vi "弹窗-提示选择Com口-30.vi"(7 "存储间隔（小时）":dbl=1.0 min=0.5, 8 "VI引用句柄":refnum<vi>, 9 "实时数据列表":refnum<vi>, 10 "测量值":cluster{"X":timestamp, "Y":dbl}[](array[cluster]), 11 "暂停发送-引用":refnum<vi>) -> (3 "存储间隔（h）":dbl=1.0 min=1.0)   [LabVIEW 2017]
uses:
  <vilib>/Utility/xml.llb/Write to XML File(string).vi
panel:
  in  "联系人数组":cluster{"姓名":string, "手机号":string}[](array[cluster])
  in  "通讯录菜单":enum16{"添加", "删除"}(ring)
  in  "确定":bool
  in  "取消":bool
  in  "选项卡控件":enum32{"通信设置", "短信通知", "调试选项"}(tab)
  in  "静音与恢复延迟（秒）":u16=1 min=1
  in  "VISA资源名称":refnum<visa-resource-name> caption="通信串口"
  in  "最大探头数":u8=1 min=1 max=32
  in  "波特率":enum16{"9600", "19200"}(ring)
  in  "检查并重置33号":bool caption="btn_微调"
  out "重置33号结果":string
  in  "密码":string
  in  "短信通道":string
  in  "员工编号":string
  in  "企业编号":string
  in  "通讯录":i32(listbox)
  in  "添加联系人":bool
  in  "探头地址":u8=1 min=1 max=1 step=1
  in  "N2":u16
  in  "N1":u16
  in  "btn_修改系数":bool
  in  "btn_微调":bool
  in  "微调大小":dbl caption="μSv/h"
  in  "微调模式":enum16{"减小", "增加"}(ring) caption="模式"
  in  "btn_改波特率":bool
  in  "修改波特率":enum16{"9600", "19200"}(ring)=enum."19200"
  # "通信信息"
  # "累积剂量"
  # "通信端口"
  # "波特率"
  # "报警静音"
  # "扫描探头数"
  # "检查隐藏探头"
  # "33号探头作为修改地址所用的临时交接地址 , 修改地址过程异常可能导致探头落入此地址 , \n1. 使用的当前通讯波特率\n2. 实时通信稳定后可设置"
  # "登录信息"
  # "通讯录"
  # "* 短信通知功能需用户自行开通，详询对接平台 http://www.c123.com/"
  # "* 通讯录表格中右键菜单添加或删除联系人"
  # "广播修改波特率"
  # "针对性修改"
  # "测量值微调（μSv/h）"
  # "计算系数"
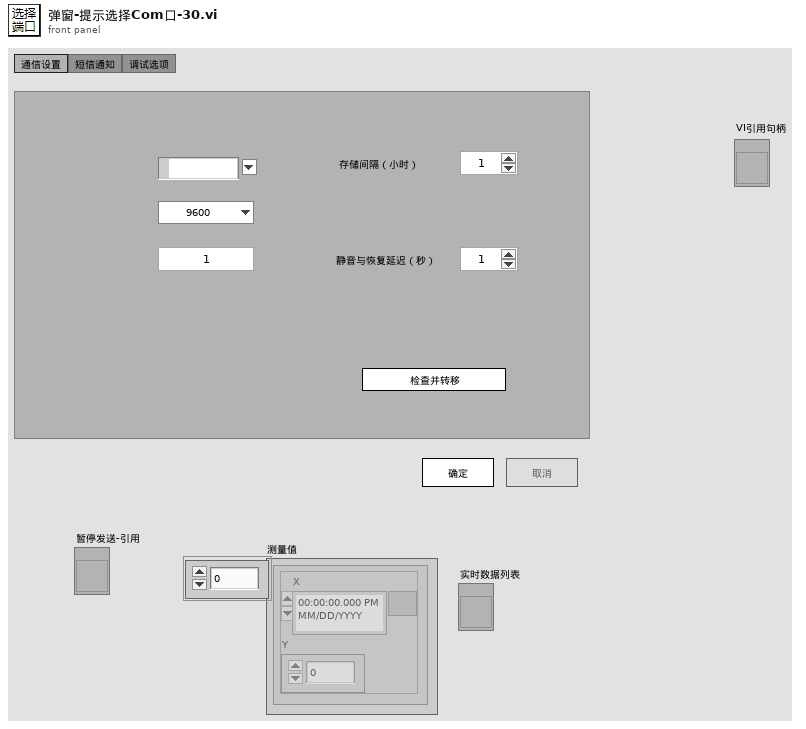
[diagram p1: front panel]
types:
  T1 = enum8{"Enabled", "Disabled", "Disabled and Grayed Out"}
  T2 = enum32{"Invalid", "Standard", "Closed", "Hidden", "Minimized", "Maximized"}
  T3 = enum32{"Page Enabled", "Page Disabled", "Page Disabled & Grayed"}
  T4 = cluster{"企业编号":string, "员工编号":string, "通道号":string, "密码":string, "联系人数组":cluster{"姓名":string, "手机号":string}[]}
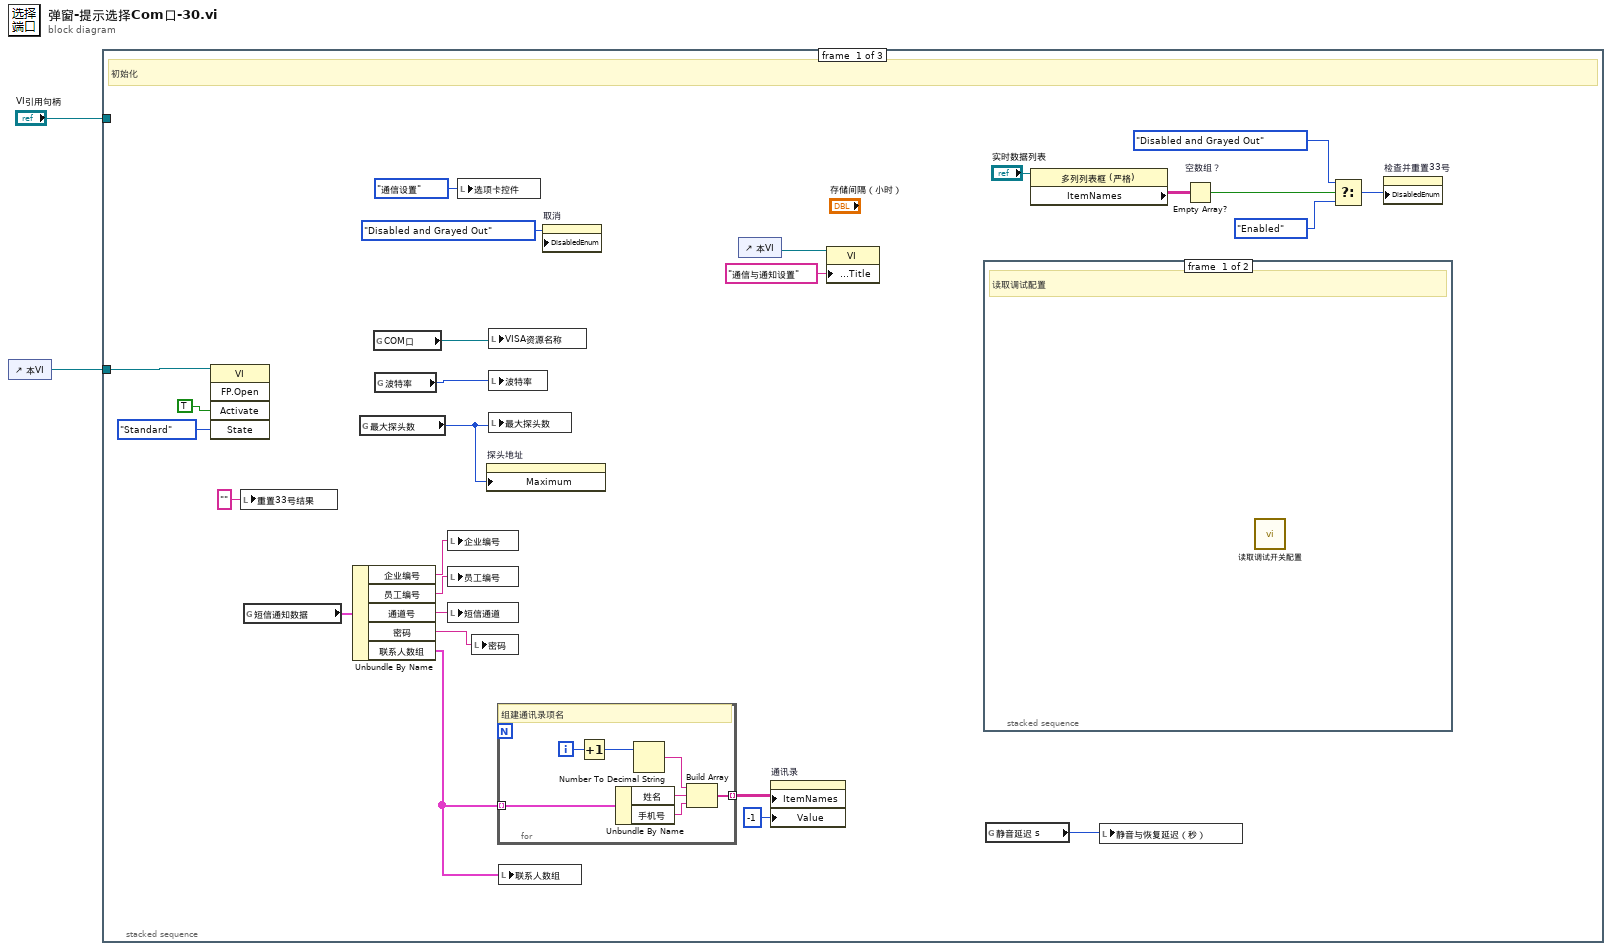
[diagram p0: block diagram]
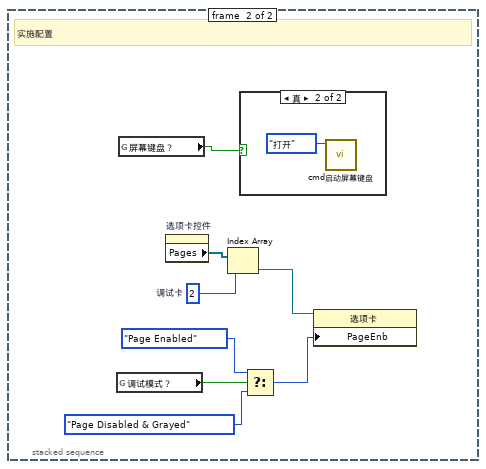
[diagram p2: hidden frame]
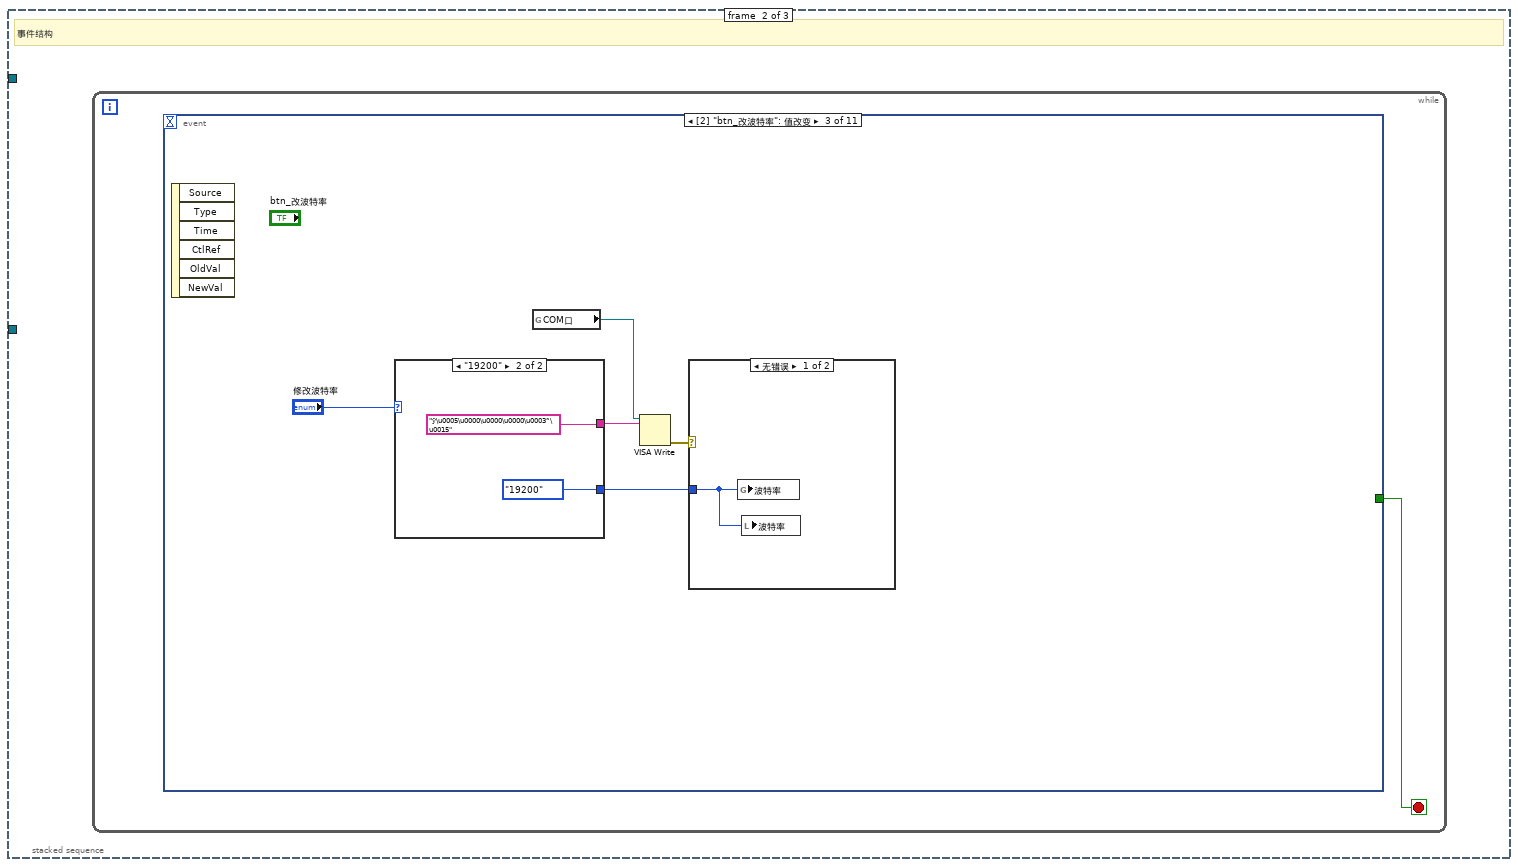
[diagram p4: hidden frame]
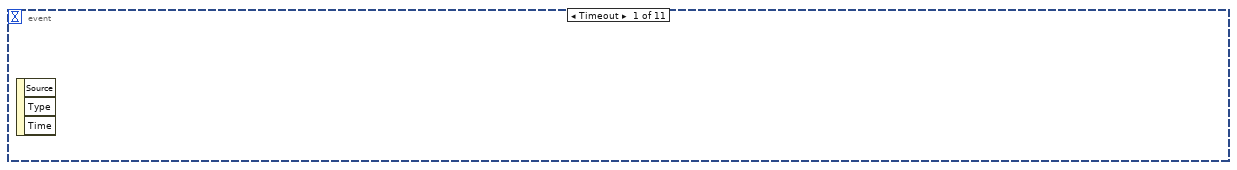
[diagram p5: hidden frame]
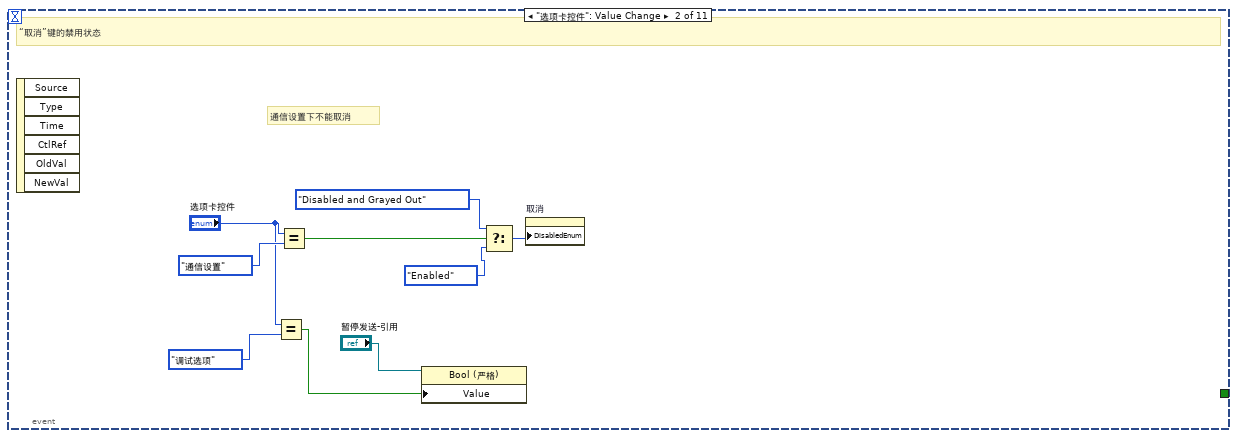
[diagram p6: hidden frame]
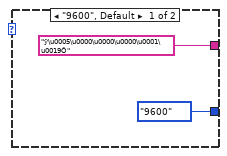
[diagram p8: hidden frame]
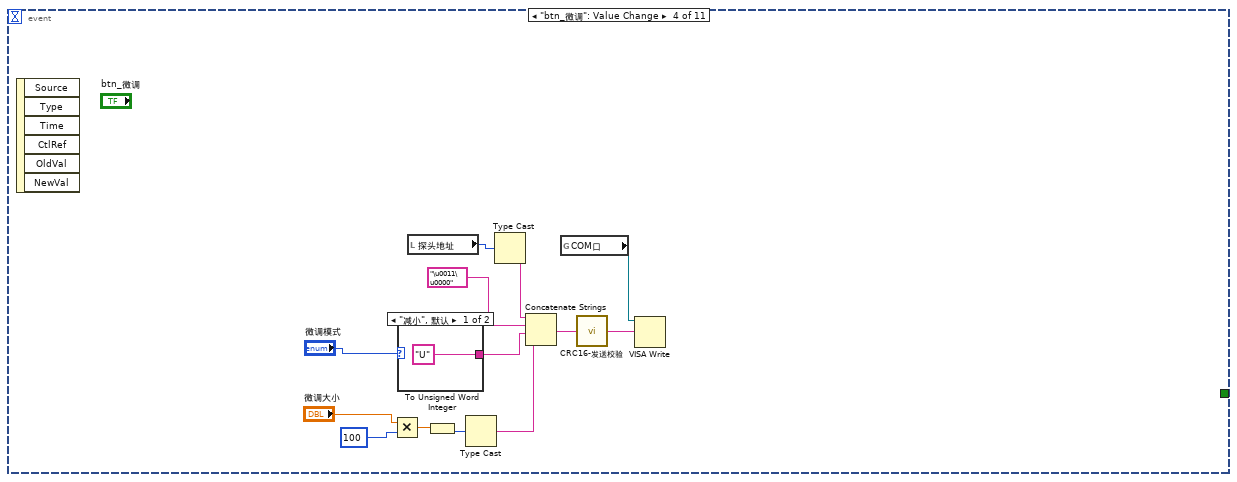
[diagram p9: hidden frame]
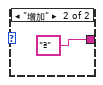
[diagram p10: hidden frame]
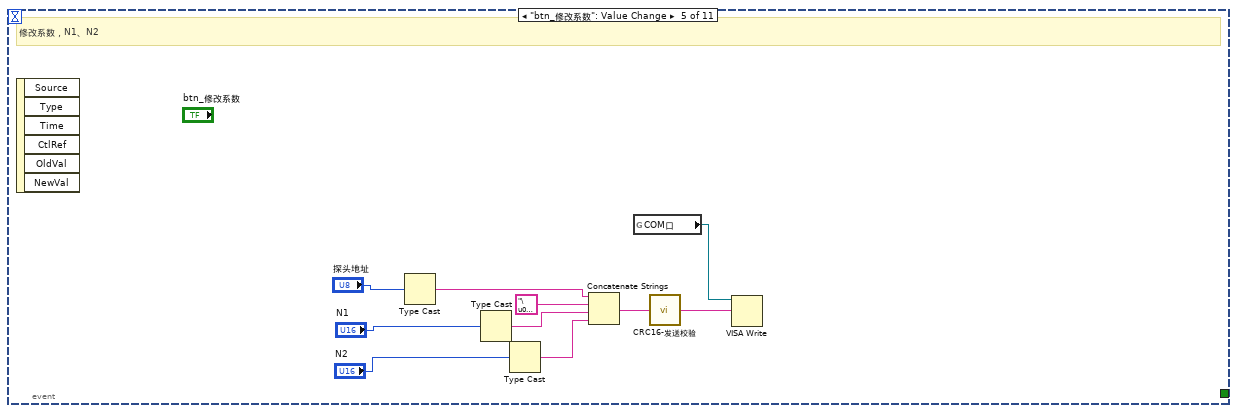
[diagram p11: hidden frame]
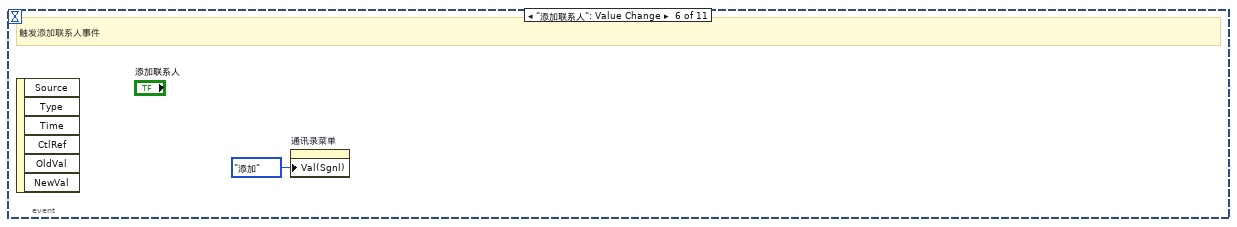
[diagram p12: hidden frame]
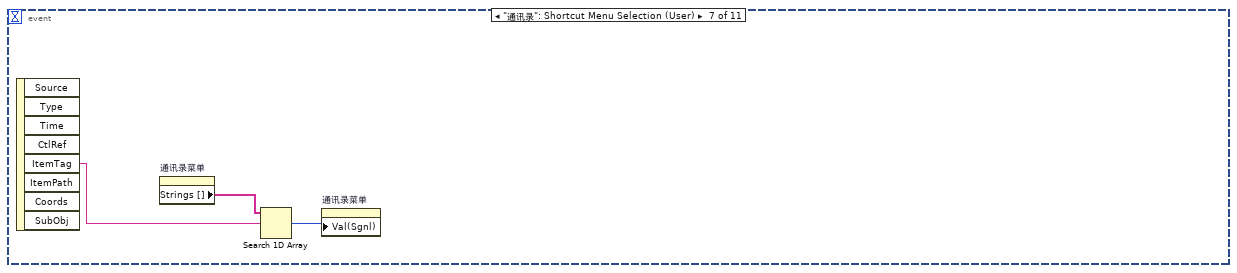
[diagram p13: hidden frame]
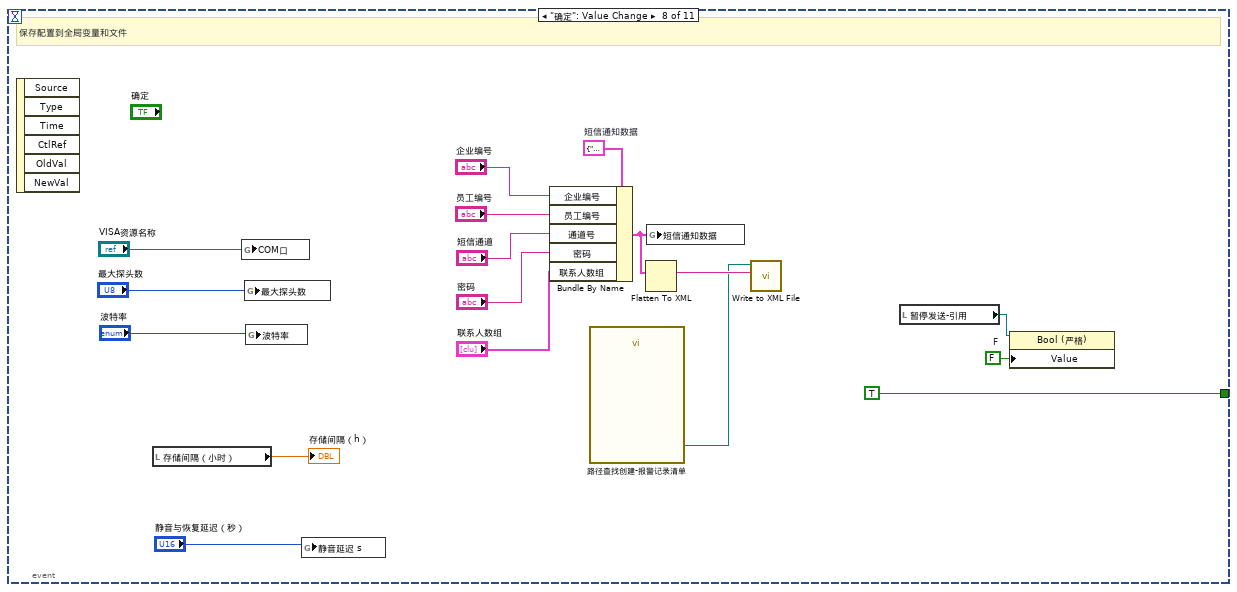
[diagram p14: hidden frame]
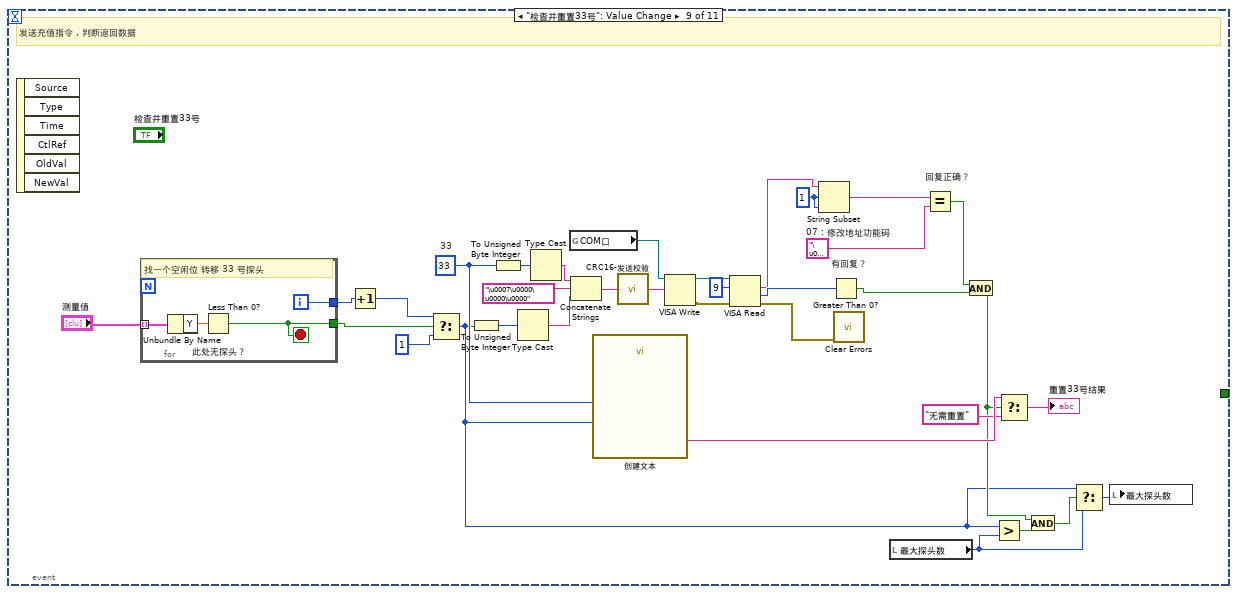
[diagram p15: hidden frame]
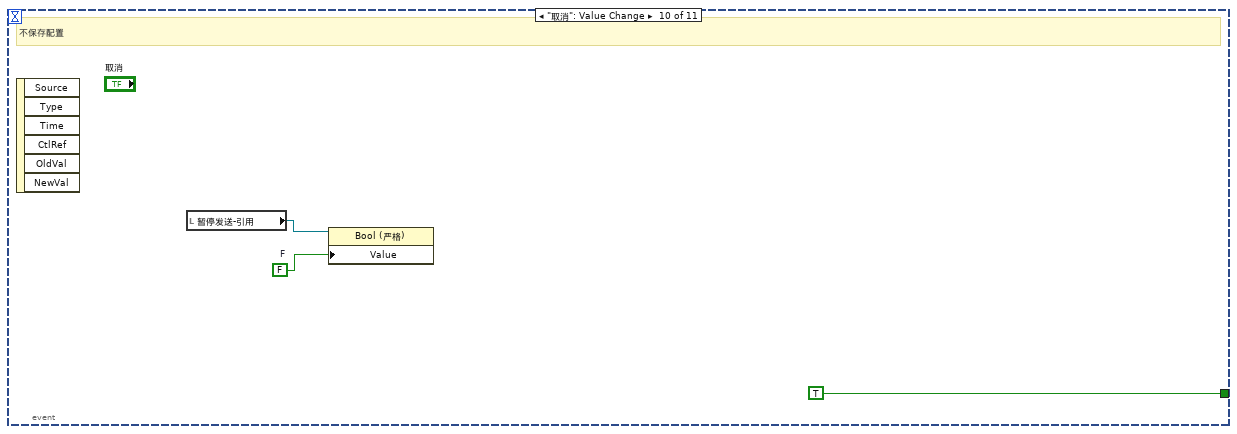
[diagram p16: hidden frame]
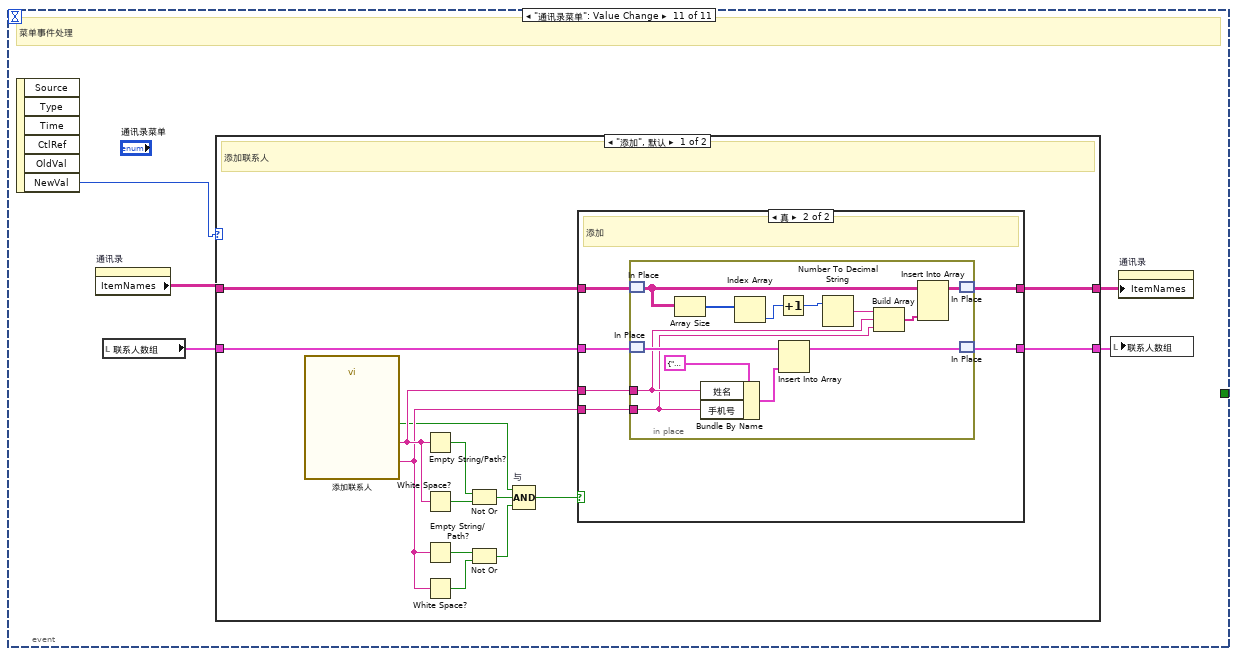
[diagram p17: hidden frame]
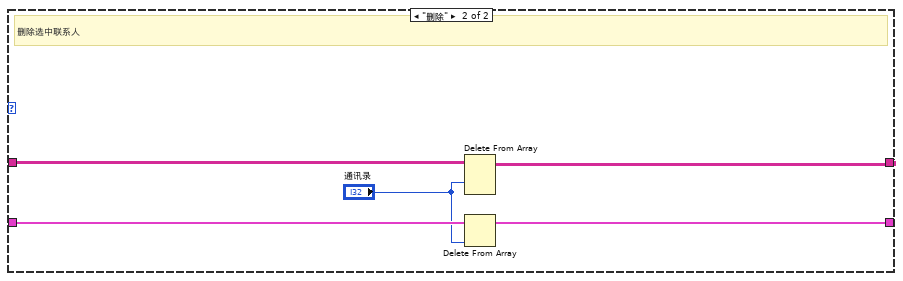
[diagram p19: hidden frame]
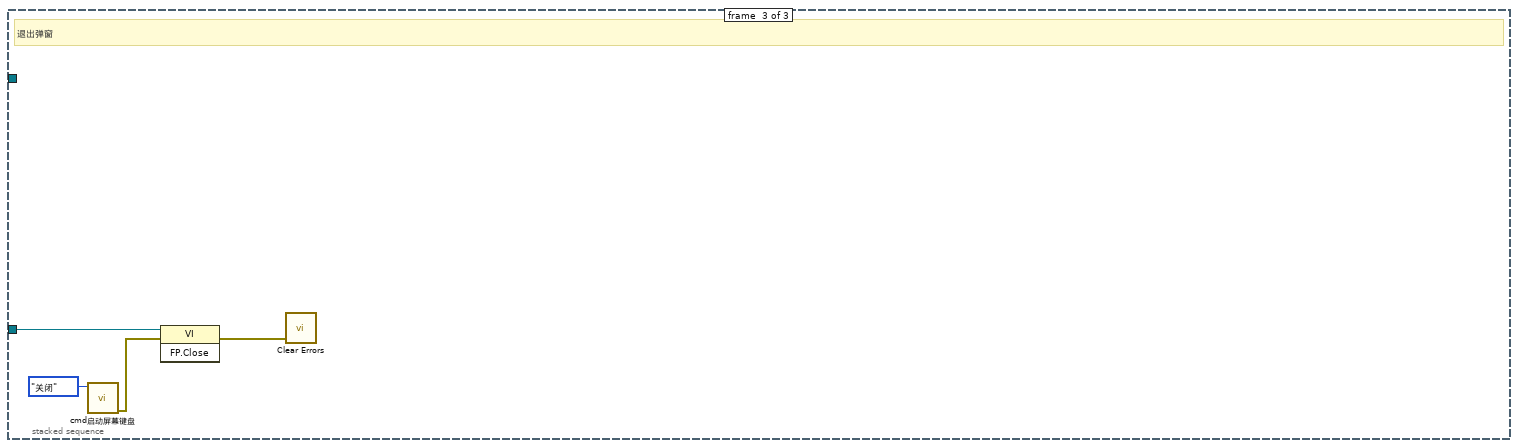
[diagram p20: hidden frame]
diagram:
  n1 = control-ref of="本VI"() -> (w1:refnum<vi>)
  n2 = stacked-sequence {
    tunnel: "VI引用句柄" -> [_ _ _]
    tunnel: w1 -> [w28 _ w200]
    frame #0 {
      # "初始化"
      n3 = invoke class="VI" method="FP.Open"(reference=w28, "Activate"=TRUE ("激活？"), "State"=T2."Standard" ("状态")) -> ()  [unwired: 2 in, 5 out]
      n4 = local write "重置33号结果"("" ("重置33号结果")) -> ()
      n5 = global read "全局变量-35点监测.vi" "短信通知数据"() -> (w19:T4)
      n6 = Unbundle By Name(w19) -> ("企业编号"=w18:string, "员工编号"=w17:string, "通道号"=w16:string, "密码"=w15:string, "联系人数组"=w14:cluster{"姓名":string, "手机号":string}[])
      n7 = global read "全局变量-35点监测.vi" "最大探头数"() -> (w11:i32)
      n8 = global read "全局变量-35点监测.vi" "COM口"() -> (w25:refnum<visa-resource-name>)
      n9 = global read "全局变量-35点监测.vi" "波特率"() -> (w24:enum16{"9600", "19200"})
      n10 = local write "企业编号"(w18) -> ()
      n11 = local write "员工编号"(w17) -> ()
      n12 = local write "短信通道"(w16) -> ()
      n13 = local write "选项卡控件"(enum32{"通信设置", "短信通知"}."通信设置" ("选项卡控件")) -> ()
      n14 = local write "密码"(w15) -> ()
      n15 = property on="探头地址" class="数字 (严格)"("Maximum"=w11) -> ()  [unwired: 2 in, 2 out]
      n16 = local write "VISA资源名称"(w25) -> ()
      n17 = local write "波特率"(w24) -> ()
      n18 = local write "最大探头数"(w11) -> ()
      n19 = for {
        tunnel: w14 -> [w44] mode=indexing
        tunnel: [w41] -> w13 mode=indexing
        i -> [w40]
        # "组建通讯录项名"
        n20 = Increment(x=w40) -> (x+1=w38:i32)
        n21 = Unbundle By Name(w44) -> ("姓名"=w43:string, "手机号"=w42:string)
        n22 = Number To Decimal String(number=w38) -> (decimal integer string=w39:string)  [unwired: 1 in]
        n23 = Build Array(w39, w43, w42) -> (w41:string[])
      }
      n24 = local write "联系人数组"(w14) -> ()
      n25 = property on="取消" class="Bool"("DisabledEnum"=T1."Disabled and Grayed Out" ("禁用")) -> ()  [unwired: 2 in, 2 out]
      n26 = control-ref of="本VI"() -> (w23:refnum<vi>)
      n27 = property on="通讯录" class="MCListbox (严格)"("ItemNames"=w13, "Value"=-1 ("通讯录")) -> ()  [unwired: 2 in, 2 out]
      n28 = property class="VI"(reference=w23, "Front Panel.Title"="通信与通知设置" ("前面板窗口:标题")) -> ()  [unwired: 1 in, 2 out]
      n29 = stacked-sequence {
        frame #0 {
          # "读取调试配置"
          n30 = call "读取调试开关配置.vi"() -> ()  [unwired: 9 in, 3 out]
        }
        frame #1 {
          w35 = 2  # 调试卡
          # "实施配置"
          n31 = global read "全局变量-35点监测.vi" "调试模式？"() -> (w33:bool)
          n32 = global read "全局变量-35点监测.vi" "屏幕键盘？"() -> (w29:bool)
          n33 = property on="选项卡控件" class="选项卡控件 (严格)"() -> ("Pages"=w36:refnum<vi>[])  [unwired: 2 in, 2 out]
          n34 = Index Array(array=w36, index=w35) -> (element=w34:refnum<vi>)
          n35 = case shown="真" w29 {
            frame False {
            }
            frame True {
              n36 = call "cmd启动屏幕键盘.vi"("软键盘开关"=enum16{"关闭", "打开"}."打开") -> ()  [unwired: 9 in, 2 out]
            }
          }
          n37 = Select(t=T3."Page Enabled" ("选项卡页启用状态"), s=w33, f=T3."Page Disabled & Grayed" ("选项卡页启用状态")) -> (s? t:f=w30:T3)
          n38 = property class="选项卡"(reference=w34, "PageEnb"=w30) -> ()  [unwired: 1 in, 2 out]
        }
      }
      n39 = global read "全局变量-35点监测.vi" "静音延迟 s"() -> (w10:u16)
      n40 = property class="多列列表框 (严格)"(reference="实时数据列表") -> ("ItemNames"=w7:string[][])  [unwired: 1 in, 2 out]
      n41 = local write "静音与恢复延迟（秒）"(w10) -> ()
      n42 = Empty Array? "空数组？"(array=w7) -> (empty?=w6:bool)
      n43 = Select(t=T1."Disabled and Grayed Out" ("禁用"), s=w6, f=T1."Enabled" ("禁用")) -> (s? t:f=w3:T1)
      n44 = property on="检查并重置33号" class="Bool"("DisabledEnum"=w3) -> ()  [unwired: 2 in, 2 out]
    }
    frame #1 {
      # "事件结构"
      n45 = while {
        stop <- w45 stop-if-true
        n46 = event shown="[2] \"btn_改波特率\": 值改变" {
          selector: _ -> [_ _ _ _ _ _ _ _ _ _ _]
          dyn-events: _ -> [_ _ _ _ _ _ _ _ _ _ _]
          timeout: _ -> [_ _ _ _ _ _ _ _ _ _ _]
          tunnel: [_ _ _ _ _ _ _ TRUE ("T") _ TRUE ("T") _] -> w45
          event Timeout {
            n47 = event-data() -> ()  [unwired: 1 in, 3 out]
          }
          event "选项卡控件": Value Change {
            # "通信设置下不能取消"
            # "“取消”键的禁用状态"
            n48 = event-data() -> ()  [unwired: 1 in, 6 out]
            n49 = Equal?(x="选项卡控件", y=enum32{"通信设置", "短信通知", "调试选项"}."调试选项" ("选项卡控件")) -> (x = y?=w46:bool)
            n50 = Equal?(x="选项卡控件", y=enum32{"通信设置", "短信通知", "调试选项"}."通信设置" ("选项卡控件")) -> (x = y?=w53:bool)
            n51 = property on="属性节点" class="Bool (严格)"(reference="暂停发送-引用", "Value"=w46) -> ()  [unwired: 1 in, 2 out]
            n52 = Select(t=T1."Disabled and Grayed Out" ("禁用"), s=w53, f=T1."Enabled" ("禁用")) -> (s? t:f=w50:T1)
            n53 = property on="取消" class="Bool"("DisabledEnum"=w50) -> ()  [unwired: 2 in, 2 out]
          }
          event "btn_改波特率": Value Change {
            n54 = event-data() -> ()  [unwired: 1 in, 6 out]
            n55 = case shown="\"19200\"" "修改波特率" {
              tunnel: ["ÿ\u0005\u0000\u0000\u0000\u0001\u0019Ô" "ÿ\u0005\u0000\u0000\u0000\u0003˜\u0015"] -> w57
              tunnel: [enum16{"9600", "19200"}."9600" ("波特率") enum16{"9600", "19200"}."19200" ("波特率")] -> w55
              frame "9600", Default {
              }
              frame "19200" {
              }
            }
            n56 = global read "全局变量-35点监测.vi" "COM口"() -> (w58:refnum<visa-resource-name>)
            n57 = VISA Write(VISA resource name=w58, write buffer=w57) -> (error out=w56:errorcluster)  [unwired: 1 in, 2 out]
            n58 = case shown="无错误" w56 {
              tunnel: w55 -> [w60 _]
              frame No Error {
                n59 = global write "全局变量-35点监测.vi" "波特率"(w60) -> ()
                n60 = local write "波特率"(w60) -> ()
              }
              frame Error {
              }
            }
          }
          event "btn_微调": Value Change {
            n61 = event-data() -> ()  [unwired: 1 in, 6 out]
            n62 = Multiply(x="微调大小", y=100) -> (x*y=w76:dbl)
            n63 = case shown="\"减小\", 默认" "微调模式" {
              tunnel: ["U" "ª"] -> w69
              frame "减小", Default {
              }
              frame "增加" {
              }
            }
            n64 = local read "探头地址"() -> (w72:u8)
            n65 = To Unsigned Word Integer(number=w76) -> (unsigned 16bit integer=w77:u16)
            n66 = Type Cast(x=w77) -> (*(type *) &x=w68:string)  [unwired: 1 in]
            n67 = Type Cast(x=w72) -> (*(type *) &x=w71:string)  [unwired: 1 in]
            n68 = Concatenate Strings(w71, "\u0011\u0000", w69, w68) -> (w67:string)
            n69 = global read "全局变量-35点监测.vi" "COM口"() -> (w65:refnum<visa-resource-name>)
            n70 = call "CRC16-发送校验.vi"("净数据"=w67) -> ("完整输出"=w66:string)
            n71 = VISA Write(VISA resource name=w65, write buffer=w66) -> ()  [unwired: 1 in, 3 out]
          }
          event "btn_修改系数": Value Change {
            # "修改系数，N1、N2"
            n72 = event-data() -> ()  [unwired: 1 in, 6 out]
            n73 = Type Cast(x="探头地址") -> (*(type *) &x=w82:string)  [unwired: 1 in]
            n74 = Type Cast(x="N1") -> (*(type *) &x=w87:string)  [unwired: 1 in]
            n75 = Type Cast(x="N2") -> (*(type *) &x=w85:string)  [unwired: 1 in]
            n76 = Concatenate Strings(w82, "\u0012", w87, w85) -> (w84:string)
            n77 = global read "全局变量-35点监测.vi" "COM口"() -> (w88:refnum<visa-resource-name>)
            n78 = call "CRC16-发送校验.vi"("净数据"=w84) -> ("完整输出"=w89:string)
            n79 = VISA Write(VISA resource name=w88, write buffer=w89) -> ()  [unwired: 1 in, 3 out]
          }
          event "添加联系人": Value Change {
            # "触发添加联系人事件"
            n80 = event-data() -> ()  [unwired: 1 in, 6 out]
            n81 = property on="通讯录菜单" class="Enum (严格)"("Val(Sgnl)"=enum16{"添加", "删除"}."添加" ("值(信号)")) -> ()  [unwired: 2 in, 2 out]
          }
          event "通讯录": Shortcut Menu Selection (User) {
            n82 = event-data() -> ("ItemTag"=w92:string)  [unwired: 1 in, 7 out]
            n83 = property on="通讯录菜单" class="Enum (严格)"() -> ("Strings []"=w93:string[])  [unwired: 2 in, 2 out]
            n84 = Search 1D Array(1D array=w93, element=w92) -> (index of element=w91:i32)  [unwired: 1 in]
            n85 = property on="通讯录菜单" class="Enum (严格)"("Val(Sgnl)"=w91) -> ()  [unwired: 2 in, 2 out]
          }
          event "确定": Value Change {
            w100 = T4 {"企业编号"="", "员工编号"="", "通道号"="", "密码"="", "联系人数组"=[]}  # 短信通知数据
            w105 = FALSE  # F
            # "保存配置到全局变量和文件"
            n86 = event-data() -> ()  [unwired: 1 in, 6 out]
            n87 = local read "存储间隔（小时）"() -> (→"存储间隔（h）":dbl)
            n88 = global write "全局变量-35点监测.vi" "COM口"("VISA资源名称") -> ()
            n89 = global write "全局变量-35点监测.vi" "最大探头数"("最大探头数") -> ()
            n90 = global write "全局变量-35点监测.vi" "波特率"("波特率") -> ()
            n91 = global write "全局变量-35点监测.vi" "静音延迟 s"("静音与恢复延迟（秒）") -> ()
            n92 = Bundle By Name(cluster=w100, "企业编号"="企业编号", "员工编号"="员工编号", "通道号"="短信通道", "密码"="密码", "联系人数组"="联系人数组") -> (w102:T4)
            n93 = call "路径查找创建-报警记录清单.vi"() -> ("短信通知配置文件"=w95:path)  [unwired: 8 in, 11 out]
            n94 = Flatten To XML(anything=w102) -> (xml string=w101:string)
            n95 = global write "全局变量-35点监测.vi" "短信通知数据"(w102) -> ()
            n96 = call-poly <vilib>:"Write to XML File.vi"("XML Input"=w101, "XML File Path"=w95) -> ()  [unwired: 7 in, 3 out]
            n97 = local read "暂停发送-引用"() -> (w106:refnum<vi>)
            n98 = property on="属性节点" class="Bool (严格)"(reference=w106, "Value"=w105) -> ()  [unwired: 1 in, 2 out]
          }
          event "检查并重置33号": Value Change {
            w120 = u8 33  # 33
            w131 = 1 ("偏移量(0)")
            w129 = "\u0007"  # 07 : 修改地址功能码
            # "发送充值指令 , 判断返回数据"
            n99 = event-data() -> ()  [unwired: 1 in, 6 out]
            n100 = for {
              tunnel: "测量值" -> [w148] mode=indexing
              tunnel: [w146] -> w124
              tunnel: [w145] -> w123
              i -> [w146]
              stop <- w145 stop-if-true
              # "找一个空闲位 转移 33 号探头"
              n101 = Unbundle By Name(w148) -> ("Y"=w147:dbl)
              n102 = Less Than 0? "此处无探头？"(x=w147) -> (x < 0?=w145:bool)
            }
            n103 = Increment(x=w124) -> (x+1=w122:i32)
            n104 = Select(t=w122, s=w123, f=1) -> (s? t:f=w113:i32)
            n105 = To Unsigned Byte Integer(number=w113) -> (unsigned 8bit integer=w136:u8)
            n106 = To Unsigned Byte Integer(number=w120) -> (unsigned 8bit integer=w135:u8)
            n107 = Type Cast(x=w136) -> (*(type *) &x=w139:string)  [unwired: 1 in]
            n108 = Type Cast(x=w135) -> (*(type *) &x=w138:string)  [unwired: 1 in]
            n109 = global read "全局变量-35点监测.vi" "COM口"() -> (w128:refnum<visa-resource-name>)
            n110 = Concatenate Strings(w138, "\u0007\u0000\u0000\u0000", w139) -> (w140:string)
            n111 = call "创建文本"("原地址"=w120, "新地址"=w113) -> ("Result"=w119:string)  [unwired: 12 in, 1 out]
            n112 = call "CRC16-发送校验.vi"("净数据"=w140) -> ("完整输出"=w143:string)
            n113 = VISA Write(VISA resource name=w128, write buffer=w143) -> (VISA resource name out=w141:refnum<visa-resource-name>, error out=w144:errorcluster)  [unwired: 1 in, 1 out]
            n114 = VISA Read(VISA resource name=w141, byte count=u32 9 ("字节总数"), error in (no error)=w144) -> (read buffer=w132:string, return count=w133:u32, error out=w134:errorcluster)  [unwired: 1 out]
            n115 = String Subset(string=w132, offset (0)=w131, length (rest)=w131) -> (substring=w130:string)
            n116 = Greater Than 0? "有回复？"(x=w133) -> (x > 0?=w127:bool)
            n117 = call <vilib>:"Clear Errors.vi"("error in (no error)"=w134) -> ()  [unwired: 5 in, 2 out]
            n118 = local read "最大探头数"() -> (w112:u8)
            n119 = Equal? "回复正确？"(x=w130, y=w129) -> (x = y?=w126:bool)
            n120 = And(x=w126, y=w127) -> (x .and. y?=w116:bool)
            n121 = Greater?(x=w113, y=w112) -> (0:w115:bool)
            n122 = Select(t=w119, s=w116, f="无需重置") -> (s? t:f=→"重置33号结果":string)
            n123 = And(x=w116, y=w115) -> (x .and. y?=w114:bool)
            n124 = Select(t=w113, s=w114, f=w112) -> (s? t:f=w111:i32)
            n125 = local write "最大探头数"(w111) -> ()
          }
          event "取消": Value Change {
            w149 = FALSE  # F
            # "不保存配置"
            n126 = event-data() -> ()  [unwired: 1 in, 6 out]
            n127 = local read "暂停发送-引用"() -> (w150:refnum<vi>)
            n128 = property on="属性节点" class="Bool (严格)"(reference=w150, "Value"=w149) -> ()  [unwired: 1 in, 2 out]
          }
          event "通讯录菜单": Value Change {
            # "菜单事件处理"
            n129 = event-data() -> ("NewVal"=w152:enum16{"添加", "删除"})  [unwired: 1 in, 5 out]
            n130 = property on="通讯录" class="MCListbox (严格)"() -> ("ItemNames"=w156:string[][])  [unwired: 2 in, 2 out]
            n131 = local read "联系人数组"() -> (w154:cluster{"姓名":string, "手机号":string}[])
            n132 = case shown="\"添加\", 默认" w152 {
              tunnel: w154 -> [w170 w196]
              tunnel: [w169 w195] -> w153
              tunnel: w156 -> [w168 w194]
              tunnel: [w167 w193] -> w155
              frame "添加", Default {
                # "添加联系人"
                n133 = call "添加联系人"() -> ("手机号码"=w165:string, "姓名"=w166:string, "确定"=w163:bool)  [unwired: 16 in, 1 out]
                n134 = Empty String/Path?(string/path=w166) -> (empty?=w162:bool)
                n135 = White Space?(1:w166) -> (0:w161:bool)
                n136 = Empty String/Path?(string/path=w165) -> (empty?=w164:bool)
                n137 = White Space?(1:w165) -> (0:w160:bool)
                n138 = Not Or(1:w161, 2:w162) -> (0:w159:bool)
                n139 = Not Or(1:w160, 2:w164) -> (0:w158:bool)
                n140 = Compound Arithmetic op=AND "与"(w163, w159, w158) -> (w157:bool)
                n141 = case shown="真" w157 {
                  tunnel: w166 -> [_ w178]
                  tunnel: w165 -> [_ w177]
                  tunnel: w170 -> [w172 w176]
                  tunnel: [w172 w175] -> w169
                  tunnel: w168 -> [w171 w174]
                  tunnel: [w171 w173] -> w167
                  frame False {
                    # "取消"
                  }
                  frame True {
                    # "添加"
                    n142 = in-place {
                      in-place-border: w178 -> [w182]
                      in-place-border: w177 -> [w181]
                      n143 = in-place-match #1(w174) -> (w186:string[][])
                      n144 = in-place-match #2(w176) -> (w191:cluster{"姓名":string, "手机号":string}[])
                      n145 = Array Size(array=w186) -> (size(s)=w185:i32[])
                      n146 = Bundle By Name(cluster=cluster{"姓名":string, "手机号":string} {"姓名"="", "手机号"=""} ("新元素/子数组"), "姓名"=w182, "手机号"=w181) -> (w187:cluster{"姓名":string, "手机号":string})
                      n147 = Index Array(array=w185) -> (element=w184:i32)  [unwired: 1 in]
                      n148 = Increment(x=w184) -> (x+1=w179:i32)
                      n149 = Insert Into Array(array=w191, new element=w187) -> (w190:cluster{"姓名":string, "手机号":string}[])  [unwired: 1 in]
                      n150 = Number To Decimal String(number=w179) -> (decimal integer string=w183:string)  [unwired: 1 in]
                      n151 = Build Array(w183, w182, w181) -> (w180:string[])
                      n152 = Insert Into Array(array=w186, new element=w180) -> (w189:string[][])  [unwired: 2 in]
                      n153 = in-place-match #1(w189) -> (w173:string[][])
                      n154 = in-place-match #2(w190) -> (w175:cluster{"姓名":string, "手机号":string}[])
                    }
                  }
                }
              }
              frame "删除" {
                # "删除选中联系人"
                n155 = Delete From Array(array=w194, index (row)="通讯录") -> (array with subset deleted=w193:string[][])  [unwired: 2 in, 1 out]
                n156 = Delete From Array(array=w196, index="通讯录") -> (array with subset deleted=w195:cluster{"姓名":string, "手机号":string}[])  [unwired: 1 in, 1 out]
              }
            }
            n157 = local write "联系人数组"(w153) -> ()
            n158 = property on="通讯录" class="MCListbox (严格)"("ItemNames"=w155) -> ()  [unwired: 2 in, 2 out]
          }
        }
      }
    }
    frame #2 {
      # "退出弹窗"
      n159 = call "cmd启动屏幕键盘.vi"("软键盘开关"=enum16{"关闭", "打开"}."关闭") -> ("error out"=w198:errorcluster)  [unwired: 9 in, 1 out]
      n160 = invoke class="VI" method="FP.Close"(reference=w200, error in=w198) -> (error out=w197:errorcluster)  [unwired: 1 in, 2 out]
      n161 = call <vilib>:"Clear Errors.vi"("error in (no error)"=w197) -> ()  [unwired: 5 in, 2 out]
    }
  }
